vi "Lowpass Filter.vi"(2 "Tf [s]":dbl, 3 "Ts [s]":dbl, 4 "Fillter input":dbl) -> (1 "Filter Output":dbl)   [LabVIEW 2022 SP3]
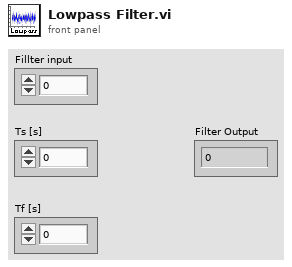
[diagram p1: front panel]
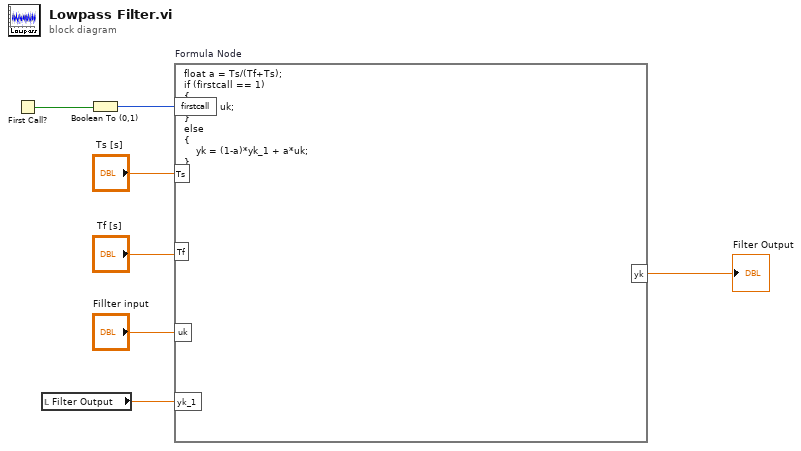
[diagram p0: block diagram]
diagram:
  n1 = First Call?() -> (First Call?: T/F=w7:bool)
  n2 = local read "Filter Output"() -> (w1:dbl)
  n3 = Boolean To (0,1)(Boolean=w7) -> (0, 1=w6:i16)
  n4 = formula code="float a = Ts/(Tf+Ts);\nif (firstcall == 1)\n{\n    yk = uk;\n}\nelse\n{\n    yk = (1-a)*yk_1 + a*uk;\n}"("firstcall"=w6, "Ts"="Ts [s]", "Tf"="Tf [s]", "uk"="Fillter input", "yk_1"=w1) -> ("yk"=→"Filter Output":dbl)
